vi "ep_Kaiser Order Estimation.vi"(6 "fs [Hz]":dbl=1.0 format="%.2f", 7 "filter type":T1, 8 "error in (no error)":errorcluster, 10 "ripple specs":T2={"passband"=0.1, "stopband"=60.0, "dB/linear? (T: dB)"=TRUE}, 11 "freq specs [Hz]":T3={"fpass 1"=0.2, "fstop 1"=0.3, "fpass 2 "=0.0, "fstop 2"=0.0}) -> (0 "error out":errorcluster, 1 "low cutoff freq [Hz]":dbl, 2 "high cutoff freq [Hz]":dbl, 3 "estimated order":i32, 4 "beta":dbl format="%.2f")   [LabVIEW 2012, in "NI_EP_Resample_Host.lvlib"]
uses:
  <vilib>/addons/Electrical Power/PQ/Resampling/NI_EP_Resample_Host.lvlib
  <vilib>/Analysis/3filter.llb/Filter Passband Type.ctl
  <vilib>/Analysis/NI_AALBase.lvlib
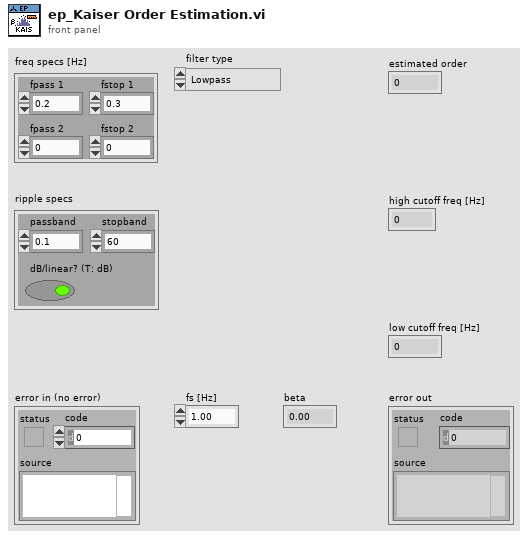
[diagram p1: front panel]
types:
  T1 = typedef "NI_AALBase.lvlib/Filter Passband Type.ctl" = enum32{"Lowpass", "Highpass", "Bandpass", "Bandstop"}
  T2 = cluster{"passband":dbl, "stopband":dbl, "dB/linear? (T: dB)":bool}
  T3 = cluster{"fpass 1":dbl, "fstop 1":dbl, "fpass 2 ":dbl, "fstop 2":dbl}
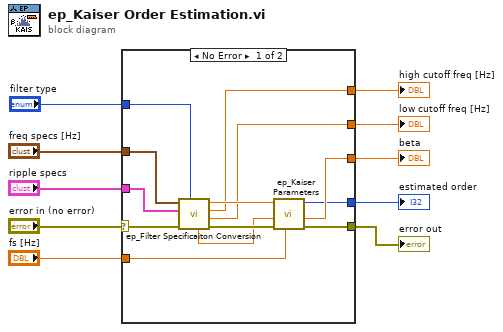
[diagram p0: block diagram]
diagram:
  n1 = case shown="No Error" "error in (no error)" {
    selector: "error in (no error)" -> [w13 w24]
    tunnel: [w11 w24] -> w10
    tunnel: [w12 _] -> w9
    tunnel: "filter type" -> [w23 _]
    tunnel: "fs [Hz]" -> [w22 _]
    tunnel: "ripple specs" -> [w14 _]
    tunnel: "freq specs [Hz]" -> [w15 _]
    tunnel: [w19 _] -> w5
    tunnel: [w17 _] -> w4
    tunnel: [w16 _] -> w3
    frame No Error {
      n2 = call <vilib>:"ep_Filter Specificaiton Conversion.vi"("filter type"=w23, "error in (no error)"=w13, "ripple specs"=w14, "freq specs [Hz]"=w15) -> ("error out"=w20:errorcluster, "low cutoff freq: fl"=w16:dbl, "high cutoff freq: fh"=w17:dbl, "min transition band"=w21:dbl, "A stop (dB)"=w18:dbl)  [unwired: 3 in]
      n3 = call <vilib>:"ep_Kaiser Parameters.vi"("fs [Hz]"=w22, "error in (no error)"=w20, "A stop [dB]"=w18, "delta f [Hz]"=w21) -> ("error out"=w11:errorcluster, "beta"=w19:dbl, "order"=w12:i32)  [unwired: 5 in]
    }
    frame Error {
    }
  }
  "error out" <- w10
  "estimated order" <- w9
  "beta" <- w5
  "high cutoff freq [Hz]" <- w4
  "low cutoff freq [Hz]" <- w3
